vi "Un-Pause Work.vi"(8 "error in (no error)":errorcluster, 11 "Process Controller in":refnum<class "Process Controller.lvclass">) -> (0 "error out":errorcluster, 3 "Process Controller out":refnum<class "Process Controller.lvclass">)   [LabVIEW 2018, in "Process Controller.lvclass"]
uses:
  Process Controller.lvclass
  C:/github/LabActor/Worker/Worker.lvclass
  C:/github/LabActor/Template Module/Template Module.lvclass
  Worker/Worker.lvclass/Worker.ctl
  NHMFL_Core/Libraries/Instruments/Instrument Driver/Worker State.ctl
  Template Module/Template Module.lvclass/Template Module.ctl
  Worker/Write Paused.vi
  Template Module/Read Reply to.vi
  Template Module/Read State.vi
  Worker/Read Paused.vi
  Worker/Write Pause requested.vi
  Worker/Read Pause requested.vi
  Template Module Messages/Result Reply Msg/Result Reply Msg.lvclass
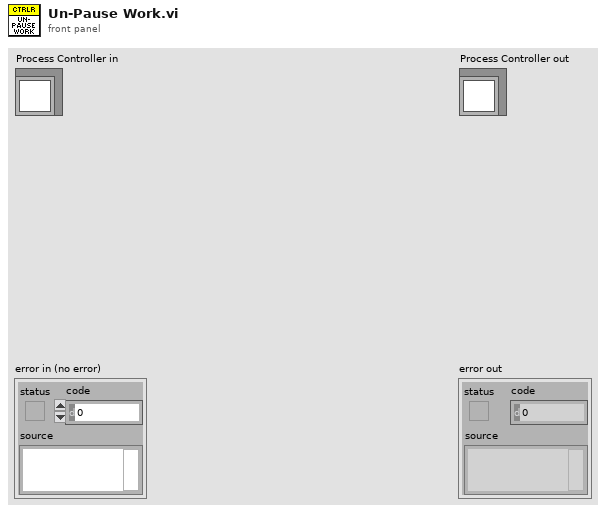
[diagram p1: front panel]
types:
  T1 = typedef "Worker State.ctl" = enum16{"Idle", "Starting", "Working", "Stopping"}
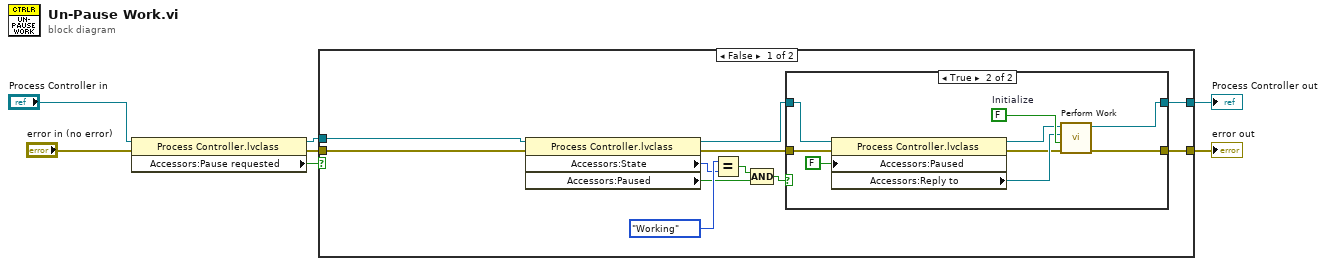
[diagram p0: block diagram]
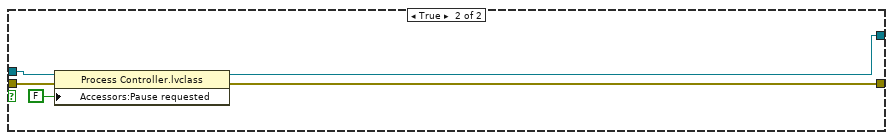
[diagram p3: hidden frame]
diagram:
  n1 = property class="Process Controller.lvclass"(reference="Process Controller in", error in="error in (no error)") -> (reference out=w2:refnum<class "Process Controller.lvclass">, error out=w4:errorcluster, "Accessors:Pause requested"=w1:bool)
  n2 = case shown="False" w1 {
    tunnel: [w11 w31] -> w6
    tunnel: [w10 w30] -> w5
    tunnel: w4 -> [w9 w33]
    tunnel: w2 -> [w8 w34]
    frame False {
      n3 = property class="Process Controller.lvclass"(reference=w8, error in=w9) -> (reference out=w13:refnum<class "Process Controller.lvclass">, error out=w12:errorcluster, "Accessors:State"=w17:T1, "Accessors:Paused"=w16:bool)
      n4 = Equal?(x=Worker_State."Working" ("State"), y=w17) -> (x = y?=w15:bool)
      n5 = Compound Arithmetic op=AND(w15, w16) -> (w14:bool)
      n6 = case shown="True" w14 {
        tunnel: w13 -> [w20 w29]
        tunnel: w12 -> [w19 w28]
        tunnel: [w19 w23] -> w11
        tunnel: [w20 w21] -> w10
        frame False {
        }
        frame True {
          w26 = FALSE  # Initialize
          n7 = property class="Process Controller.lvclass"(reference=w29, error in=w28, "Accessors:Paused"=FALSE ("Pause requested")) -> (reference out=w22:refnum<class "Process Controller.lvclass">, error out=w24:errorcluster, "Accessors:Reply to"=w25:refnum<class "Result Reply Msg.lvclass">)
          n8 = call-dynamic "Perform Work.vi"("error in (no error)"=w24, "Initialize"=w26, "Reply to"=w25, "Measure Controller in"=w22) -> ("error out"=w23:errorcluster, "Measure Controller out"=w21:refnum<class "Process Controller.lvclass">)  [unwired: 6 in]
        }
      }
    }
    frame True {
      n9 = property class="Process Controller.lvclass"(reference=w34, error in=w33, "Accessors:Pause requested"=FALSE ("Pause requested")) -> (reference out=w30:refnum<class "Process Controller.lvclass">, error out=w31:errorcluster)
    }
  }
  "error out" <- w6
  "Process Controller out" <- w5
